vi "ExcelToDB_ErrorQty.vi"() -> ()   [LabVIEW 2012]
uses:
  <vilib>/Utility/NIReport.llb/NI_report.lvclass
  <vilib>/addons/database/Connection.llb/DB Tools Open Connec (Path).vi
  <vilib>/Utility/NIReport.llb/Excel/NI_Excel.lvclass
  <vilib>/addons/database/NI_Database_API.lvlib
panel:
  out "error out 4":errorcluster
  in  "Cluster":T1
  out "error out 3":errorcluster
  in  "start cell":string="a2"
  out "error out":errorcluster
  in  "template (empty)":path=path "O:/Monitor/NVT/MachineQtyCheckList.xls"
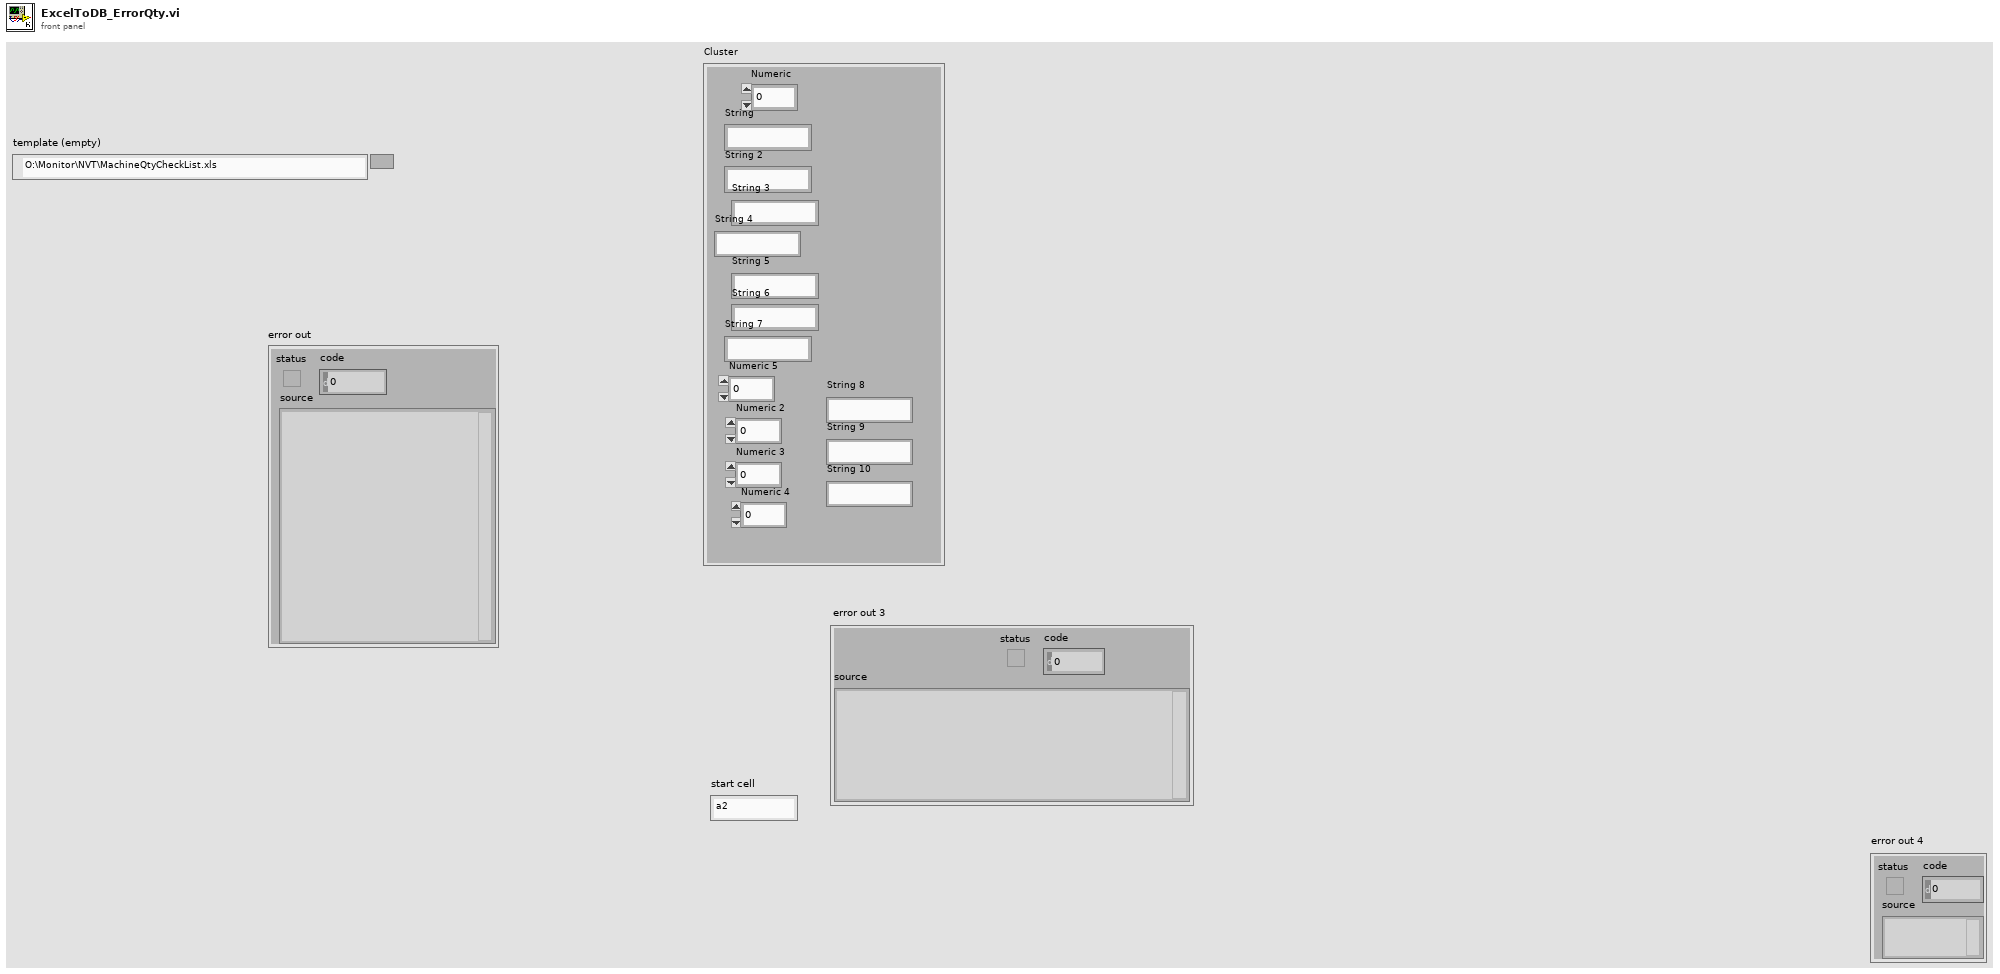
[diagram p1: front panel]
types:
  T1 = cluster{"Numeric":dbl, "String":string, "String 2":string, "String 3":string, "String 4":string, "String 5":string, "String 6":string, "String 7":string, "Numeric 5":dbl, "Numeric 2":dbl, "Numeric 3":dbl, "Numeric 4":dbl, "String 8":string, "String 9":string, "String 10":string}
  T2 = enum16{"Standard Report", "HTML", "Word", "Excel"}
  T3 = typedef "NI_Database_API.lvlib/Conn ObjectReference.ctl" = refnum<k1>
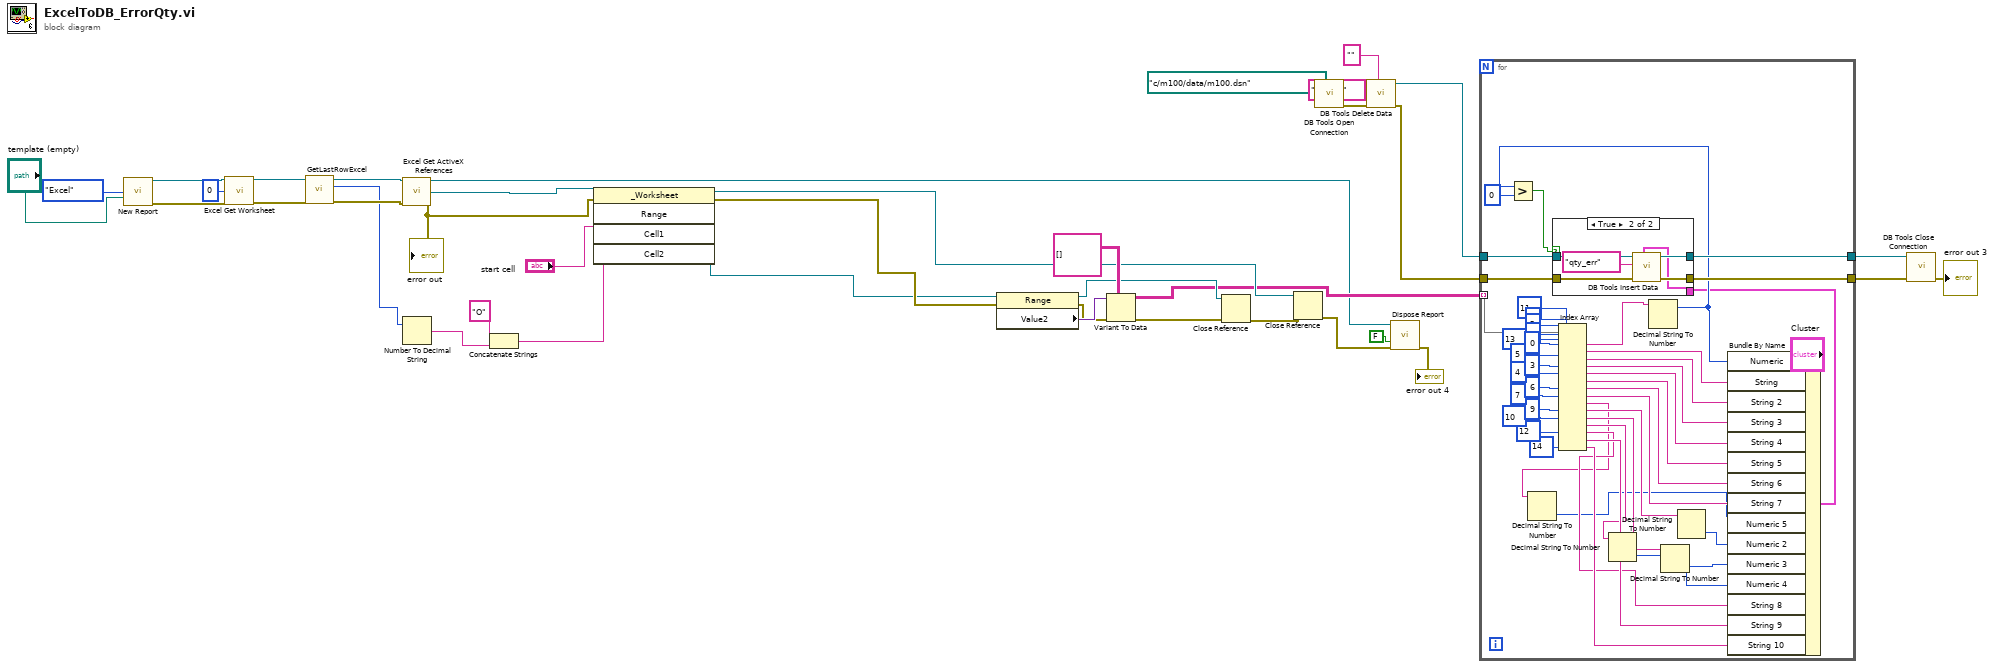
[diagram p0: block diagram]
diagram:
  n1 = call <vilib>:"New Report.vi"("report type"=T2."Excel", "template (empty)"="template (empty)") -> ("report out"=w38:refnum<class "NI_report.lvclass">, "error out"=w37:errorcluster)  [unwired: 12 in]
  n2 = call <vilib>:"Excel Get Worksheet.vi"("report in"=w38, "worksheet index (0)"=0, "error in (no error)"=w37) -> ("report out"=w18:refnum<class "NI_report.lvclass">, "error out"=w17:errorcluster)  [unwired: 11 in]
  n3 = call "GetLastRowExcel.vi"("error in (no error)"=w17, "report in"=w18) -> ("error out"=w15:errorcluster, "row"=w14:i32, "report out"=w16:refnum<class "NI_report.lvclass">)  [unwired: 7 in]
  n4 = call <vilib>:"Excel Get ActiveX References.vi"("report in"=w16, "error in (no error)"=w15) -> ("report out"=w7:refnum<class "NI_report.lvclass">, "Excel._Worksheet"=w34:refnum<k7>, "error out"=w19:errorcluster)  [unwired: 7 in, 4 out]
  "error out" <- w19
  n5 = Number To Decimal String(number=w14) -> (decimal integer string=w12:string)  [unwired: 1 in]
  n6 = Concatenate Strings("O" ("string"), w12) -> (w11:string)
  n7 = invoke class="_Worksheet" method="Range"(reference=w34, error in=w19, "Cell1"="start cell", "Cell2"=w11) -> (reference out=w26:refnum<k7>, error out=w31:errorcluster, "Range"=w30:refnum<k7>)  [unwired: 1 in, 2 out]
  n8 = property class="Range"(reference=w30, error in=w31) -> (reference out=w27:refnum<k7>, error out=w32:errorcluster, "Value2"=w33:variant)
  n9 = Variant To Data(error in=w32, type=string[][] [], Variant=w33) -> (data=w20:string[][], error out=w28:errorcluster)
  n10 = Close Reference(reference=w27, error in (no error)=w28) -> (error out=w25:errorcluster)
  n11 = Close Reference(reference=w26, error in (no error)=w25) -> (error out=w8:errorcluster)
  n12 = call-poly <vilib>:"DB Tools Open Connection.vi"("connection information"=path "c:/m100/data/m100.dsn") -> ("error out"=w6:errorcluster, "connection reference"=w5:T3)  [unwired: 7 in]
  n13 = call <vilib>:"DB Tools Delete Data.vi"("condition"="", "error in (no error)"=w6, "table"="qty_err", "connection reference"=w5) -> ("error out"=w3:errorcluster, "connection reference out"=w4:T3)  [unwired: 6 in]
  n14 = call-dynamic "Dispose Report.vi"("report in"=w7, "save changes? (F)"=FALSE, "error in (no error)"=w8) -> ("error out"=→"error out 4":errorcluster)  [unwired: 12 in]
  n15 = for {
    tunnel: w4 -> [w84]
    tunnel: w3 -> [w83]
    tunnel: [w82] -> w22
    tunnel: [w81] -> w21
    tunnel: w20 -> [w80] mode=indexing
    n16 = Index Array(array=w80, index #1=0 ("index"), index #2=1 ("index"), index #3=2 ("index"), index #4=3 ("index"), index #5=4 ("index"), index #6=5 ("index"), index #7=6 ("index"), index #8=7 ("index"), index #9=8 ("index"), index #10=9 ("index"), index #11=10 ("index"), index #12=11 ("index"), index #13=12 ("index"), index #14=13 ("index"), index #15=14 ("index")) -> (element #1=w65:string, element #2=w64:string, element #3=w63:string, element #4=w62:string, element #5=w61:string, element #6=w60:string, element #7=w59:string, element #8=w58:string, element #9=w46:string, element #10=w47:string, element #11=w48:string, element #12=w49:string, element #13=w50:string, element #14=w51:string, element #15=w52:string)
    n17 = Decimal String To Number(string=w46) -> (number=w45:i32)  [unwired: 2 in, 1 out]
    n18 = Decimal String To Number(string=w49) -> (number=w42:i32)  [unwired: 2 in, 1 out]
    n19 = Decimal String To Number(string=w65) -> (offset past number=w57:i32)  [unwired: 2 in, 1 out]
    n20 = Greater?(x=w57, y=0) -> (0:w55:bool)
    n21 = Decimal String To Number(string=w48) -> (number=w41:i32)  [unwired: 2 in, 1 out]
    n22 = Decimal String To Number(string=w47) -> (number=w43:i32)  [unwired: 2 in, 1 out]
    n23 = Bundle By Name(cluster="Cluster", "Numeric"=w57, "String"=w64, "String 2"=w63, "String 3"=w62, "String 4"=w61, "String 5"=w60, "String 6"=w59, "String 7"=w58, "Numeric 5"=w45, "Numeric 2"=w43, "Numeric 3"=w41, "Numeric 4"=w42, "String 8"=w50, "String 9"=w51, "String 10"=w52) -> (w44:T1)
    n24 = case shown="True" w55 {
      tunnel: w84 -> [w86 w91]
      tunnel: w83 -> [w85 w90]
      tunnel: [w86 w89] -> w82
      tunnel: [w85 w88] -> w81
      tunnel: w44 -> [_ w87]
      frame False {
      }
      frame True {
        n25 = call <vilib>:"DB Tools Insert Data.vi"("data"=w87, "error in (no error)"=w90, "table"="qty_err", "connection reference"=w91) -> ("error out"=w88:errorcluster, "connection reference out"=w89:T3)  [unwired: 6 in]
      }
    }
  }
  n26 = call <vilib>:"DB Tools Close Connection.vi"("error in (no error)"=w21, "connection reference"=w22) -> ("error out"=→"error out 3":errorcluster)  [unwired: 5 in]
